vi "populateILCMapWithFA.vi"(8 "error in (no error)":errorcluster, 11 "ILCCommunications in":refnum<class "ILCCommunications.lvclass">) -> (0 "error out":errorcluster, 3 "ILCCommunications out":refnum<class "ILCCommunications.lvclass">)   [LabVIEW 2016, in "ILCCommunications.lvclass"]
uses:
  ILCCommunications.lvclass
  ILCCommunications.lvclass/ILCCommunications.ctl
  DataTypes/General/ILCMap.ctl
  DataTypes/General/ILCTypes.ctl
  Common_RT_ILC/ILC/ILC.lvclass/ILC.ctl
  Common_RT_FAILC/FAILC/FAILC.lvclass
  D:/Code/ts_M1M3Support/Common_RT_ILC/ILC/ILC.lvclass
  DataTypes/General/M1M3SupportGeneral.lvlib
  Common_RT_ILC/ILC/ILC.lvclass
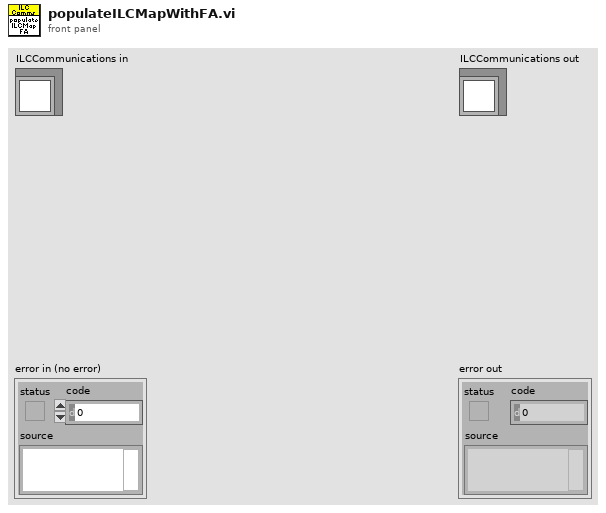
[diagram p1: front panel]
types:
  T1 = typedef "M1M3SupportGeneral.lvlib/ILCMap.ctl" = cluster{"Index":i32, "Type":T2}
  T2 = typedef "M1M3SupportGeneral.lvlib/ILCTypes.ctl" = enum16{"Hardpoint", "Force"}
  T3 = typedef "RTILC.lvlib/ILCData.ctl" = cluster{"Constants":T4, "Command":T5, "Telemetry":T7, "Responses":T8, "Timestamps":T10, "Timings":T11}
  T4 = typedef "RTILC.lvlib/ILCConstants.ctl" = cluster{"Subnet":u8, "Address":u8}
  T5 = typedef "RTILC.lvlib/ILCCommand.ctl" = cluster{"Mode":u16, "TemporaryAddress":u8, "ADCScanRate":T6, "ADCChannel":u8, "ADCOffset":sgl, "ADCSensitivity":sgl}
  T6 = typedef "RTILC.lvlib/ILCScanRates.ctl" = u8
  T7 = typedef "RTILC.lvlib/ILCTelemetry.ctl" = cluster{"UniqueID":u64, "FirmwareType":u8, "NetworkNodeType":u8, "ILCOption":u8, "NetworkNodeOption":u8, "MajorRevision":u8, "MinorRevision":u8, "FirmwareName":string, "Mode":u16, "MajorFault":bool, "MinorFault":bool, "FaultOverride":bool, "MainCalibrationError":bool, "BackupCalibrationError":bool, "UniqueIDCRCMismatch":bool, "AppTypeNodeTypeMismatch":bool, "AppMissing":bool, "AppCRCMismatch":bool, "TEDSNotFound":bool, "TEDS1Mismatch":bool, "TEDS2Mismatch":bool, "WatchdogResetDetected":bool, "BrownoutDetected":bool, "EventTrapResetDetected":bool, "MotorPowerFault":bool, "SSRPowerFault":bool, "AuxPowerFault":bool, "SMCPowerFault":bool, "TemporaryAddress":u8, "ADCScanRate":T6, "MainADCCalibrationK":sgl[], "MainSensorOffset":sgl[], "MainSensorSensitivity":sgl[], "BackupADCCalibrationK":sgl[], "BackupSensorOffset":sgl[], "BackupSensorSensitivity":sgl[]}
  T8 = typedef "RTILC.lvlib/ILCResponses.ctl" = cluster{"ReportServerID":T9, "ReportServerStatus":T9, "Mode":T9, "TemporaryAddress":T9, "Reset":T9, "ADCScanRate":T9, "ADCOffsetSensitivity":T9, "ReportCalibrationData":T9}
  T9 = typedef "RTModbus.lvlib/ExceptionCodes.ctl" = u16
  T10 = typedef "RTILC.lvlib/ILCTimestamps.ctl" = cluster{"ReportServerID":dbl, "ReportServerStatus":dbl, "Mode":dbl, "TemporaryAddress":dbl, "Reset":dbl, "ADCScanRate":dbl, "ADCOffsetSensitivity":dbl, "ReportCalibrationData":dbl}
  T11 = typedef "RTILC.lvlib/ILCTimings.ctl" = cluster{"ReportServerID":u32, "ReportServerStatus":u32, "Mode":u32, "TemporaryAddress":u32, "Reset":u32, "ADCScanRate":u32, "ADCOffsetSensitivity":u32, "ReportCalibrationData":u32}
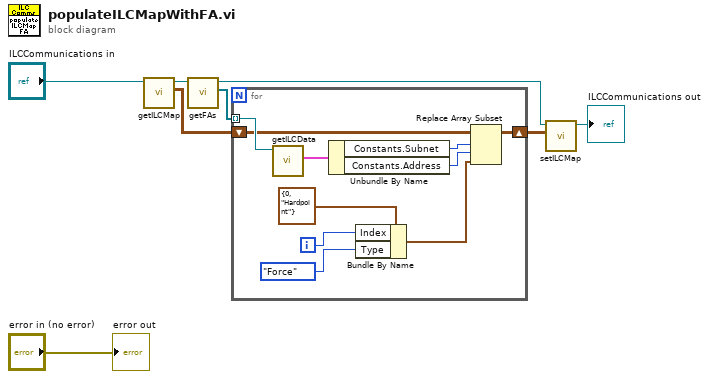
[diagram p0: block diagram]
diagram:
  n1 = call "getILCMap.vi"("ILCCommunications in"="ILCCommunications in") -> ("ILCMap"=w6:T1[][], "ILCCommunications out"=w3:refnum<class "ILCCommunications.lvclass">)  [unwired: 9 in]
  n2 = call "getFAs.vi"("ILCCommunications in"=w3) -> ("FAs"=w1:refnum<class "FAILC.lvclass">[], "ILCCommunications out"=w2:refnum<class "ILCCommunications.lvclass">)  [unwired: 9 in]
  n3 = for {
    tunnel: w1 -> [w18] mode=indexing
    shift-right: [w9] -> w5
    shift-left: w6 -> [w16]
    i -> [w12]
    n4 = call "getILCData.vi"("ILC in"=w18) -> ("ILCData"=w17:T3)  [unwired: 9 in, 1 out]
    n5 = Unbundle By Name(w17) -> ("Constants.Subnet"=w15:u8, "Constants.Address"=w14:u8)
    n6 = Bundle By Name(cluster=T1 {"Index"=0, "Type"=enum."Hardpoint"} ("new element/subarray"), "Index"=w12, "Type"=ILCTypes."Force") -> (w10:T1)
    n7 = Replace Array Subset(array=w16, new element=w10, index (row)=w15, index (col)=w14) -> (w9:T1[][])
  }
  n8 = call "setILCMap.vi"("ILCMap"=w5, "ILCCommunications in"=w2) -> ("ILCCommunications out"=→"ILCCommunications out":refnum<class "ILCCommunications.lvclass">)  [unwired: 9 in]
  "error out" <- "error in (no error)"
